vi "Read VI path.vi"(8 "error in":errorcluster, 11 "UI Reference configuration in":refnum<class "io configuration.lvclass">) -> (0 "error out":errorcluster, 2 "VI path":path, 3 "UI Reference configuration out":refnum<class "io configuration.lvclass">)   [LabVIEW 2015, in "io configuration.lvclass"]
uses:
  io configuration.lvclass
  io configuration.lvclass/io configuration.ctl
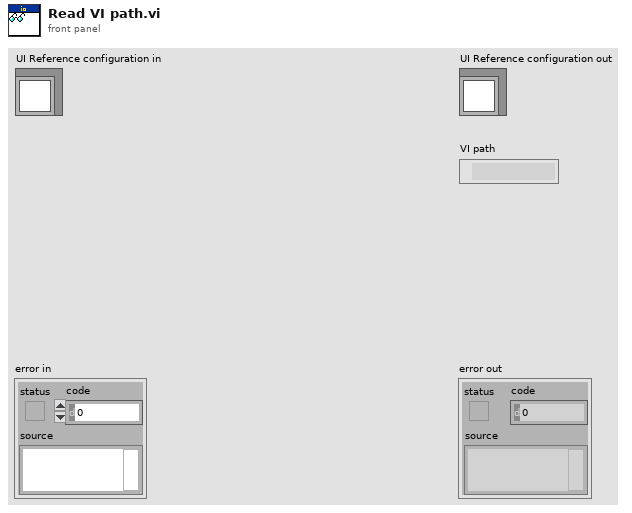
[diagram p1: front panel]
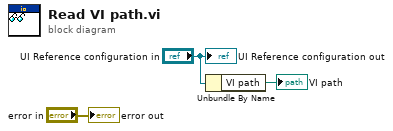
[diagram p0: block diagram]
diagram:
  n1 = Unbundle By Name("UI Reference configuration in") -> ("VI path"=→"VI path":path)
  "error out" <- "error in"
  "UI Reference configuration out" <- "UI Reference configuration in"
